vi "Aligning flash.vi"(11 "Thing 1":bool) -> (3 "Flashy the LED":bool)   [LabVIEW 2011]
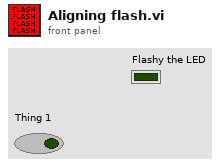
[diagram p1: front panel]
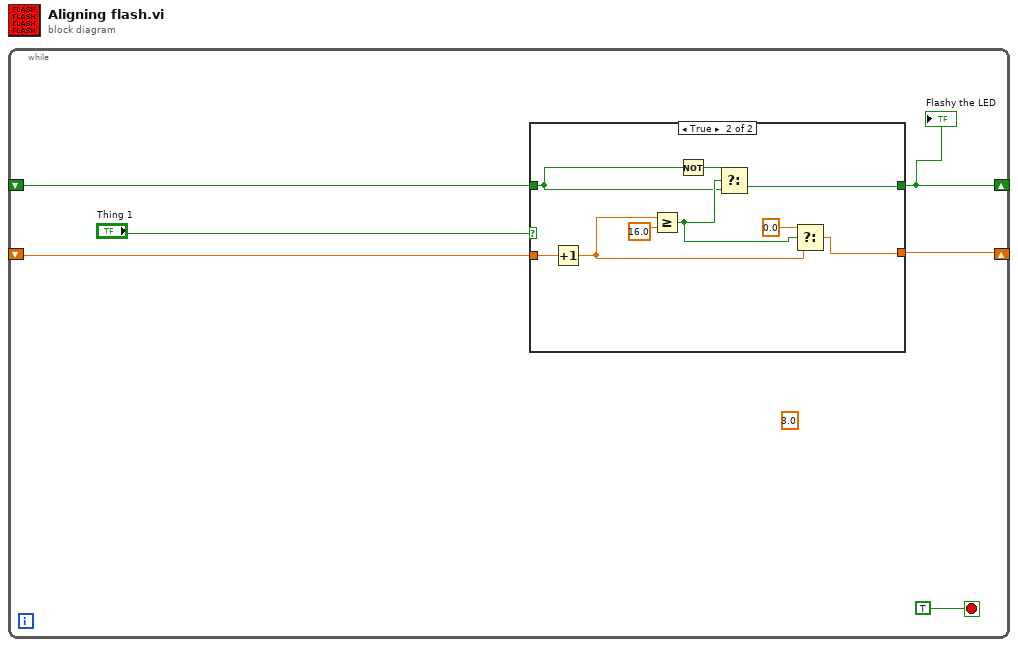
[diagram p0: block diagram]
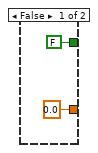
[diagram p2: hidden frame]
diagram:
  (unwired) 3.0 ("y")
  n1 = while {
    shift-right: [w5] -> _
    shift-left: _ -> [w6]
    shift-right: [w2] -> _
    shift-left: _ -> [w4]
    stop <- TRUE stop-if-true
    n2 = case shown="True" "Thing 1" {
      tunnel: w6 -> [_ w17]
      tunnel: [0.0 ("t") w16] -> w5
      tunnel: [FALSE ("Latched") w9] -> w2
      tunnel: w4 -> [_ w10]
      frame False {
      }
      frame True {
        n3 = Increment(x=w17) -> (x+1=w13:dbl)
        n4 = Greater Or Equal?(x=w13, y=16.0) -> (x >= y?=w11:bool)
        n5 = Not(x=w10) -> (.not. x?=w12:bool)
        n6 = Select(t=w12, s=w11, f=w10) -> (s? t:f=w9:bool)
        n7 = Select(t=0.0, s=w11, f=w13) -> (s? t:f=w16:dbl)
      }
    }
    "Flashy the LED" <- w2
  }
